vi "Actualizar Refrescos y Papas.vi"(11 "Cluster Producto":T1) -> ()   [LabVIEW 2019, in "REFRESCOS Y PAPAS ACTOR.lvlib" / "REFRESCOS Y PAPAS ACTOR.lvclass"]
uses:
  REFRESCOS Y PAPAS ACTOR.lvclass
  <vilib>/Utility/config.llb/Write Key (I32).vi
  <vilib>/Utility/config.llb/NI_LVConfig.lvlib
panel:
  in  "REFRESCOS Y PAPAS ACTOR in":refnum<class "REFRESCOS Y PAPAS ACTOR.lvclass">
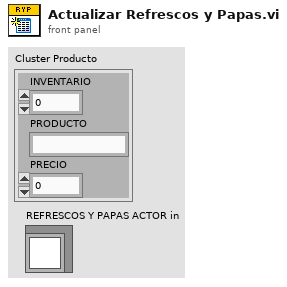
[diagram p1: front panel]
types:
  T1 = cluster{"INVENTARIO":i32, "PRODUCTO":string, "PRECIO":dbl}
  T2 = typedef "NI_LVConfig.lvlib/Config Data RefNum.ctl" = refnum<k1>
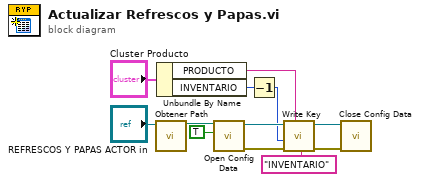
[diagram p0: block diagram]
diagram:
  n1 = call "Obtener Path.vi"("REFRESCOS Y PAPAS ACTOR in"="REFRESCOS Y PAPAS ACTOR in") -> ("appended path"=w12:path)  [unwired: 10 in]
  n2 = Unbundle By Name("Cluster Producto") -> ("PRODUCTO"=w3:string, "INVENTARIO"=w2:i32)
  n3 = call <vilib>:"Open Config Data.vi"("create file if necessary (T)"=TRUE, "configuration file path"=w12) -> ("error out"=w9:errorcluster, "refnum"=w10:T2)  [unwired: 7 in, 1 out]
  n4 = Decrement(x=w2) -> (x-1=w1:i32)
  n5 = call-poly <vilib>:"Write Key.vi"("section"=w3, "error in (no error)"=w9, "value"=w1, "key"="INVENTARIO", "refnum"=w10) -> ("error out"=w8:errorcluster, "refnum out"=w7:T2)  [unwired: 4 in, 1 out]
  n6 = call <vilib>:"Close Config Data.vi"("error in (no error)"=w8, "refnum"=w7) -> ()  [unwired: 8 in, 2 out]
